vi "Sorting Data new.vi"(5 "Clusters in":T1, 6 "error in (no error)":errorcluster, 8 "Data in":string="\u0000\f)ÒîD\u0000\u001b\u001bI÷éˆ’þÿ\u0005\u0001\u0000\u0000\u0001k\u0000\u0000\u0000d\u0002\u0005\u0000\u001e\u0000\u0000\u0001\u0001\u0001\u0002\u0002\u0001\u0002\u0002\u0002\u0003\u0002\u0004\u0002\u0005\u0003=\u0005\u0001\u0005\u0002\u0005\u0003\u0005\u0004\u0005\u0005ÿÿ\u0002\u0001\u0000\u000b\u0000\u0000S7-400 CP\u0000\u0002\u0002\u0000\t\u0000\u0000pn-io-1\u0000\u0002\u0003\u0000\u0006\u0000\u0000\u0000*\u0002\u0001\u0002\u0004\u0000\u0004\u0000\u0000\u0002\u0000\u0001\u0002\u0000\u000e\u0000\u0001À¨dVÿÿÿ\u0000\u0000\u0000\u0000\u0000") -> (0 "error out":errorcluster, 4 "Clusters out":T1)   [LabVIEW 2017]
uses:
  TypeDefs/DCP and LLDP Cluster.ctl
  TypeDefs/DCP ARRAY.ctl
  TypeDefs/Profinet Ident.ctl
  TypeDefs/LLDP ARRAY.ctl
  TypeDefs/LLDP.ctl
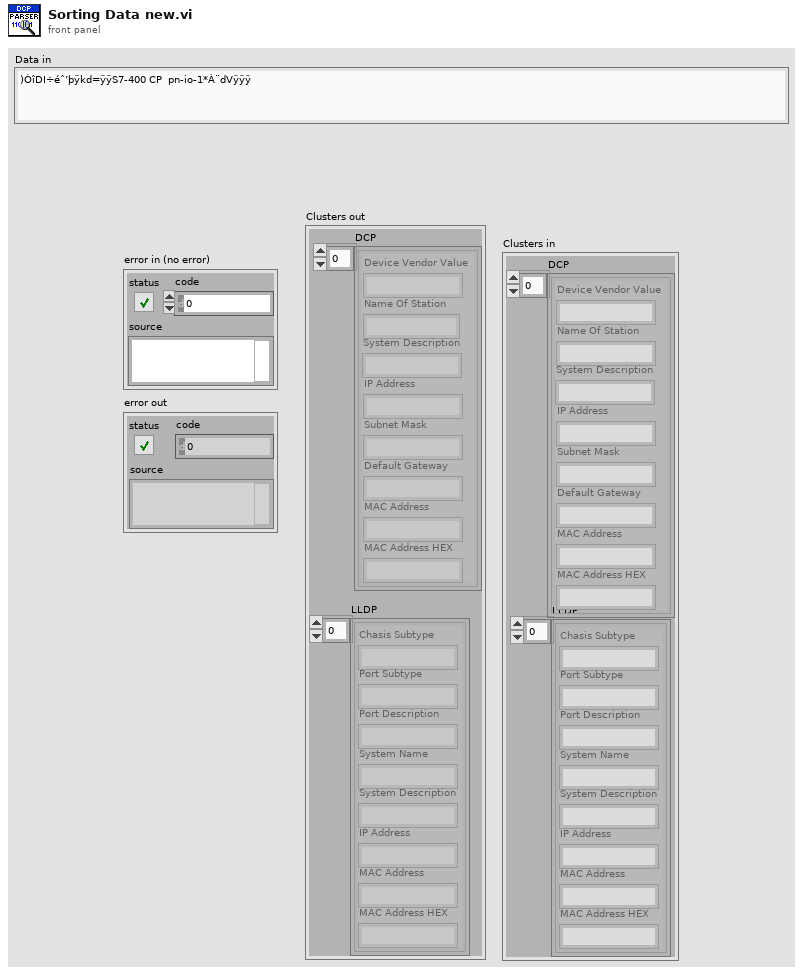
[diagram p1: front panel]
types:
  T1 = typedef "DCP and LLDP Cluster.ctl" = cluster{"DCP":T2, "LLDP":T4}
  T2 = typedef "DCP ARRAY.ctl" = T3[]
  T3 = typedef "Profinet Ident.ctl" = cluster{"Device Vendor Value":string, "Name Of Station":string, "IP Address":string, "Subnet Mask":string, "Default Gateway":string, "MAC Address":string, "MAC Address HEX":string, "System Description ":string}
  T4 = typedef "LLDP ARRAY.ctl" = T5[]
  T5 = typedef "LLDP.ctl" = cluster{"Chasis Subtype":string, "Port Subtype":string, "Port Description":string, "System Name":string, "System Description":string, "IP Address":string, "MAC Address":string, "MAC Address HEX":string}
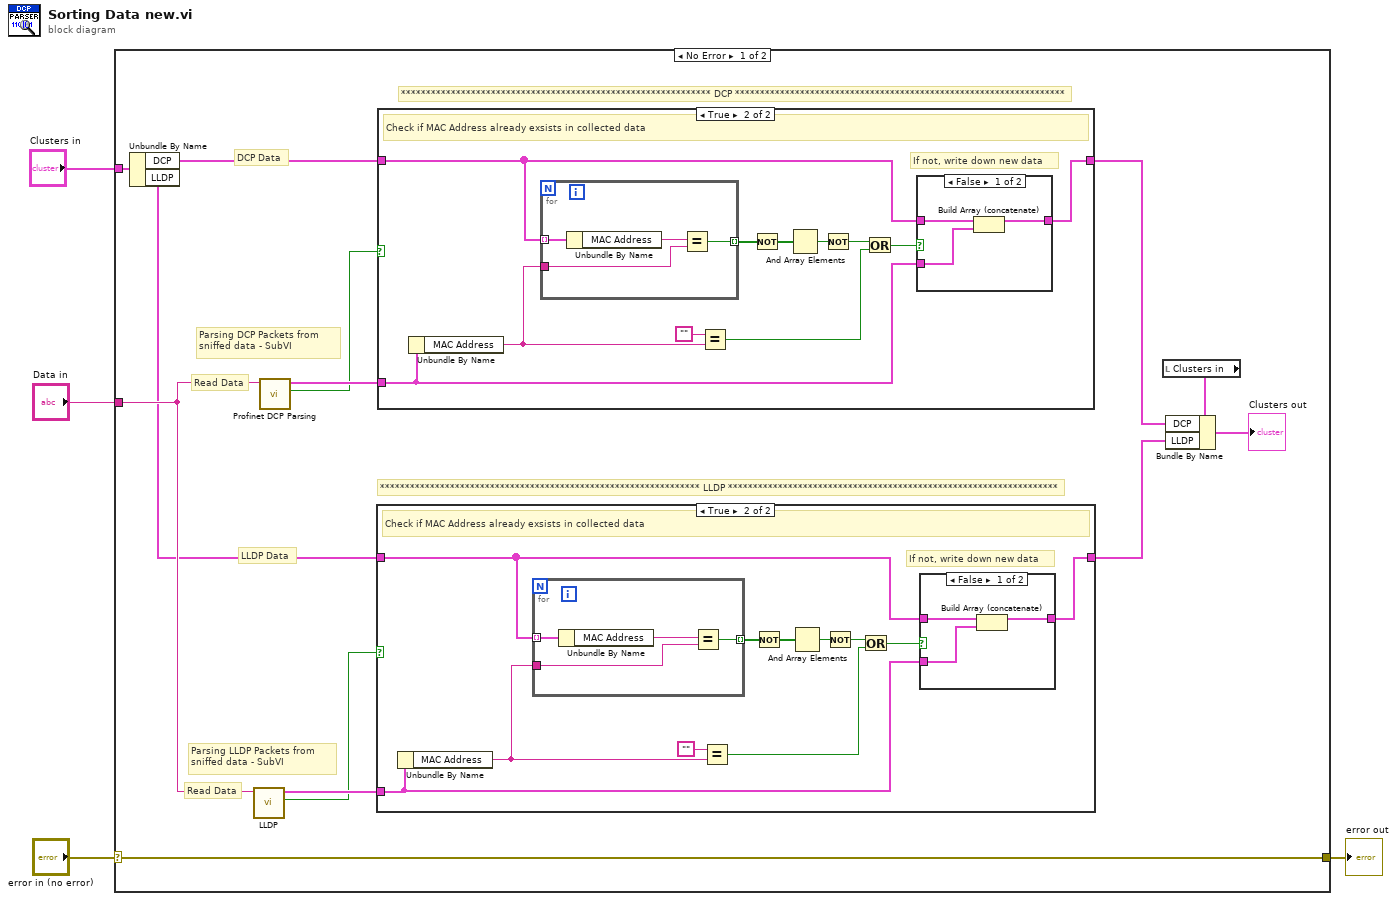
[diagram p0: block diagram]
diagram:
  n1 = case shown="No Error" "error in (no error)" {
    selector: "error in (no error)" -> [w16 w58]
    tunnel: "Data in" -> [w17 _]
    tunnel: "Clusters in" -> [w7 _]
    tunnel: [w16 w58] -> w1
    frame No Error {
      # "Read Data"
      # "Read Data"
      # "LLDP Data"
      # "DCP Data"
      # "Parsing LLDP Packets from \nsniffed data - SubVI"
      # "Parsing DCP Packets from \nsniffed data - SubVI"
      # "************************************************************** DCP ******************************************************************"
      # "**************************************************************** LLDP ******************************************************************"
      n2 = Unbundle By Name(w7) -> ("DCP"=w13:T2, "LLDP"=w12:T4)
      n3 = call "LLDP.vi"("Data in"=w17) -> ("LLDP packet"=w8:bool, "LLDP"=w15:T5)  [unwired: 8 in]
      n4 = call "Profinet DCP Parsing.vi"("Data in"=w17) -> ("PROFINET DCP Response"=w9:bool, "Profinet Ident"=w14:T3)  [unwired: 9 in]
      n5 = case shown="True" w8 {
        tunnel: w15 -> [_ w21]
        tunnel: w12 -> [w18 w20]
        tunnel: [w18 w19] -> w10
        frame False {
          # "Do nothing - read packet is not a LLDP packet"
        }
        frame True {
          # "If not, write down new data"
          # "Check if MAC Address already exsists in collected data"
          n6 = Unbundle By Name(w21) -> ("MAC Address"=w24:string)
          n7 = for {
            tunnel: w20 -> [w33] mode=indexing
            tunnel: [w32] -> w26 mode=indexing
            tunnel: w24 -> [w31]
            n8 = Unbundle By Name(w33) -> ("MAC Address"=w30:string)
            n9 = Equal?(x=w30, y=w31) -> (x = y?=w32:bool)
          }
          n10 = Equal?(x="", y=w24) -> (x = y?=w22:bool)
          n11 = Not(x=w26) -> (.not. x?=w27:bool[])
          n12 = And Array Elements(Boolean array=w27) -> (logical AND=w28:bool)
          n13 = Not(x=w28) -> (.not. x?=w23:bool)
          n14 = Or(x=w23, y=w22) -> (x .or. y?=w29:bool)
          n15 = case shown="False" w29 {
            tunnel: [w36 w37] -> w19
            tunnel: w21 -> [w35 _]
            tunnel: w20 -> [w34 w37]
            frame False {
              n16 = Build Array (concatenate)(w34, w35) -> (w36:T4)
            }
            frame True {
            }
          }
        }
      }
      n17 = case shown="True" w9 {
        tunnel: w14 -> [_ w41]
        tunnel: w13 -> [w38 w40]
        tunnel: [w38 w39] -> w11
        frame False {
          # "Do nothing - read packet is not a DCP packet"
        }
        frame True {
          # "If not, write down new data"
          # "Check if MAC Address already exsists in collected data"
          n18 = Unbundle By Name(w41) -> ("MAC Address"=w44:string)
          n19 = for {
            tunnel: w40 -> [w53] mode=indexing
            tunnel: [w52] -> w46 mode=indexing
            tunnel: w44 -> [w51]
            n20 = Unbundle By Name(w53) -> ("MAC Address"=w50:string)
            n21 = Equal?(x=w50, y=w51) -> (x = y?=w52:bool)
          }
          n22 = Equal?(x="", y=w44) -> (x = y?=w42:bool)
          n23 = Not(x=w46) -> (.not. x?=w47:bool[])
          n24 = And Array Elements(Boolean array=w47) -> (logical AND=w48:bool)
          n25 = Not(x=w48) -> (.not. x?=w43:bool)
          n26 = Or(x=w43, y=w42) -> (x .or. y?=w49:bool)
          n27 = case shown="False" w49 {
            tunnel: [w56 w57] -> w39
            tunnel: w41 -> [w55 _]
            tunnel: w40 -> [w54 w57]
            frame False {
              n28 = Build Array (concatenate)(w54, w55) -> (w56:T2)
            }
            frame True {
            }
          }
        }
      }
      n29 = local read "Clusters in"() -> (w6:T1)
      n30 = Bundle By Name(cluster=w6, "DCP"=w11, "LLDP"=w10) -> (→"Clusters out":T1)
    }
    frame Error {
    }
  }
  "error out" <- w1
